vi "Compressor With Cylinder.vi"() -> ()   [LabVIEW 2013]
doc: "Compressor with Cylinder \n\nThis example shows how to control a compressor, extend and retract a cylinder, and optionally use a limit switch to retract automatically.\n\nThis example works with the NI 9403 module connected to a Digital Sidecar. The Digital Sidecar should have 12V applied to the WAGO connector. A SPIKE relay is used to turn the compressor on and off. The PWM type input on the SPIKE should be wired to RELAY 1 on the Digital Sidecar. The GND and 12V inputs on the SPIKE should get power from the battery through a 20A fuse on the Power Distribution Board. The M+ and M- outputs from the SPIKE should be wired to the compressor. Wire M+ to the red compressor wire, and M- to the black compressor wire. The Pressure Switch is wired to DIGITAL I/O 1. This input determines when the SPIKE relay gets energized to run the compressor. The Limit Switch is wired to DIGITAL I/O 2. It causes the cylinder to retract when the Auto Retract button is pressed.\n\nThis example also uses the Solenoid Breakout connected to the NI 9472 to control the SMC double solenoid valve. From the Solenoid Breakout, channel 1 is wired to terminal A on the valve, and channel 2 is wired to terminal B on the valve.\n\nRefer to the Pneumatics Manual for air connections. Your pneumatics setup should include a compressor, pressure switch, tank, regulator, valve, flow controls, cylinder, plug valve, etc.\n\nTo run this example you should have a pneumatic system with air pressure connected to the P input on the SMC double solenoid valve. The A output of the valve should be connected via a flow control to the backend of a cylinder. The B output of the valve should be connected via a flow control to the frontend of a cylinder. When the cylinder is extended, it should physically depress the Limit Switch.\n\nWith the VI running, pressing the Extend button will push the cylinder shaft out, and pressing the Retract button will pull it back. Notice that the Extend and Retract buttons have their Mechanical Action set to Latch When Pressed. This means they stay pressed (ON) until they are read by the program, then they return to the OFF position. This works because once the SMC solenoid valve is pulled one direction, it stays in that position until it is pulled in the opposite direction - it only needs to be momentarily energized. The Auto Retract button can be used to make the cylinder return automatically. With the Auto Retract button ON, pressing the Extend button will push the cylinder out, and it will retract when it hits the limit switch."
uses:
  <vilib>/Rock Robotics/WPI/Solenoid/WPI_SolenoidChannel.ctl
  <vilib>/Rock Robotics/SystemInterfaces/DIO/FPGA_DIOChannel.ctl
  <vilib>/Rock Robotics/SystemInterfaces/DIO/FPGA_DIORelayChannel.ctl
  <vilib>/Rock Robotics/SystemInterfaces/Typedef/FPGA_TypedefDigitalModule.ctl
  <vilib>/Rock Robotics/SystemInterfaces/Typedef/FPGA_TypedefSolenoidModule.ctl
  <vilib>/Rock Robotics/WPI/Solenoid/WPI_SolenoidValue.ctl
  <vilib>/Rock Robotics/WPI/Solenoid/WPI_SolenoidOpenDouble.vi
  <vilib>/Rock Robotics/WPI/Solenoid/WPI_SolenoidSetEnum.vi
panel:
  in  "CylinderAction":T1
  out "Compressor Running?":bool
  in  "Solenoid Module":T2
  out "Cylinder Limit":bool
  in  "Limit Switch Channel":T3=enum."DIO 2"
  in  "Retract Solenoid Channel":T4=enum."Solenoid 2"
  in  "Switch and Relay Module":T5
  in  "RelayChannel":T6
  in  "Pressure Switch Channel":T3
  in  "Extend Solenoid Channel":T4
  out "Compressor Enabled?":bool
  in  "stop":bool
  # "Set these inputs before running."
  # "These can be set while running."
  # "Output information."
  # "Wiring Diagram for Digital Sidecar connected to an NI 9403"
  # "when extended, the cylinder should depress this"
  # "Limit\nSwitch"
  # "(-)"
  # "B"
  # "A"
  # "8\n7\n6\n5\n4\n3\n2\n1"
  # "RELAY"
  # "Pressure\nSwitch"
  # "Connect\nPower\nHere"
  # "GND"
  # "M-"
  # "Connect\nCompressor\nHere"
  # "SPIKE"
  # "12V"
  # "M+"
  # "B"
  # "20A"
  # "fuse"
  # "SPIKE Relay"
  # "PWM cable"
  # "COM"
  # "NC"
  # "NO"
  # "NC"
  # "C"
  # "PWR"
  # "SIG"
  # "(-)"
  # "14\n13\n12\n11\n10\n9\n8\n7\n6\n5\n4\n3\n2\n1"
  # "DIGITAL I/O"
  # "Digital Sidecar"
  # "Wiring Diagram for Solenoid Breakout connected to an NI 9472"
  # "GND"
  # "SIG"
  # "8\n7\n6\n5\n4\n3\n2\n1"
  # "+"
  # "12V from\nbattery"
  # "-"
  # "tubing port for retract side of cylinder"
  # "tubing port for extend side of cylinder"
  # "\"power good\"\n  LED"
  # "SMC double solenoid valve"
  # "B"
  # "A"
  # "B"
  # "A"
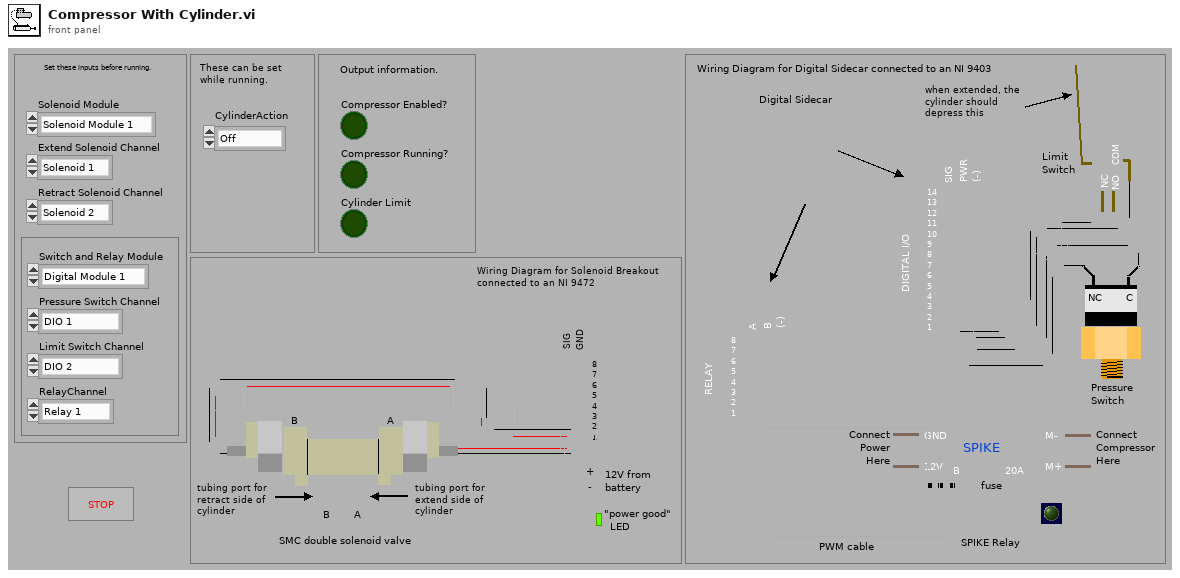
[diagram p1: front panel]
types:
  T1 = typedef "WPI_SolenoidValue.ctl" = enum16{"Off", "On", "Forward", "Reverse"}
  T2 = typedef "FPGA_TypedefSolenoidModule.ctl" = enum16{"Solenoid Module 1", "Solenoid Module 2"}
  T3 = typedef "FPGA_DIOChannel.ctl" = enum8{"DIO 1", "DIO 2", "DIO 3", "DIO 4", "DIO 5", "DIO 6", "DIO 7", "DIO 8", "DIO 9", "DIO 10", "DIO 11", "DIO 12", "DIO 13", "DIO 14", "Invalid"}
  T4 = typedef "WPI_SolenoidChannel.ctl" = enum8{"Solenoid 1", "Solenoid 2", "Solenoid 3", "Solenoid 4", "Solenoid 5", "Solenoid 6", "Solenoid 7", "Solenoid 8", "Invalid"}
  T5 = typedef "FPGA_TypedefDigitalModule.ctl" = enum16{"Digital Module 1", "Digital Module 2"}
  T6 = typedef "FPGA_DIORelayChannel.ctl" = enum8{"Relay 1", "Relay 2", "Relay 3", "Relay 4", "Relay 5", "Relay 6", "Relay 7", "Relay 8", "Invalid"}
  T7 = typedef "WPI_CompressorDevRef.ctl" = cluster{"DevStatus":errorcluster, "DigitalInputDevRef":T8, "RelayDevRef":T9}
  T8 = typedef "WPI_DigitalInputDevRef.ctl" = cluster{"DevStatus":errorcluster, "DIO Channel":T3, "Digital Module":T5}
  T9 = typedef "WPI_RelayDevRef.ctl" = cluster{"DevStatus":errorcluster, "Relay Channel":T6, "Digital Module":T5, "Relay Direction":T10}
  T10 = typedef "WPI_RelayDirection.ctl" = enum16{"Both directions", "Forward only", "Reverse only"}
  T11 = typedef "WPI_SolenoidDevRef.ctl" = cluster{"DevStatus":errorcluster, "Solenoid Module":T2, "Forward Solenoid Channel":T4, "Reverse Solenoid Channel":T4}
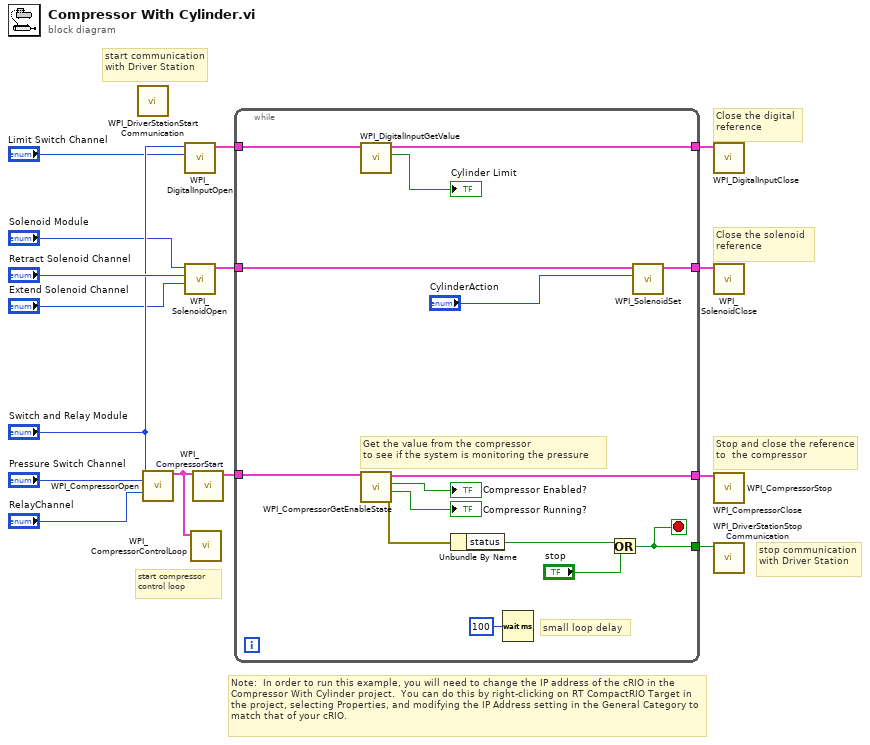
[diagram p0: block diagram]
diagram:
  # "start compressor control loop"
  # "Close the digital\nreference"
  # "Close the solenoid\nreference"
  # "stop communication with Driver Station"
  # "start communication with Driver Station"
  # "Note:  In order to run this example, you will need to change the IP address of the cRIO in the Compressor With Cylinder project.  You can do this by right-clicking on RT CompactRIO Target in the project, selecting Properties, and modifying the IP Address setting in the General Category to match that of your cRIO."
  # "Stop and close the reference to  the compressor"
  n1 = call <vilib>:"WPI_DriverStationStart Communication.vi"() -> ()  [unwired: 1 in, 11 out]
  n2 = call <vilib>:"WPI_CompressorOpen.vi"("Pressure Switch Digital Module (Module 1)"="Switch and Relay Module", "Pressure Switch DIO Channel"="Pressure Switch Channel", "Relay Channel"="RelayChannel") -> ("CompressorDevRef"=w1:T7)  [unwired: 2 in, 10 out]
  n3 = call <vilib>:"WPI_DigitalInputOpen.vi"("DIO Channel"="Limit Switch Channel", "Digital Module (Module 1)"="Switch and Relay Module") -> ("DigitalInputDevRef"=w7:T8)  [unwired: 1 in, 8 out]
  n4 = call-poly <vilib>:"WPI_SolenoidOpen.vi"("Reverse Solenoid Channel"="Extend Solenoid Channel", "Forward Solenoid Channel"="Retract Solenoid Channel", "Solenoid Module (Module 1)"="Solenoid Module") -> ("SolenoidDevRef"=w9:T11)  [unwired: 1 in, 7 out]
  n5 = call <vilib>:"WPI_CompressorControlLoop.vi"("CompressorDevRef"=w1) -> ()  [unwired: 11 in]
  n6 = call <vilib>:"WPI_CompressorStart.vi"("CompressorDevRef"=w1) -> ("CompressorDevRef"=w15:T7)  [unwired: 1 in, 9 out]
  n7 = while {
    tunnel: w15 -> [w31]
    tunnel: [w30] -> w14
    tunnel: [w28] -> w11
    tunnel: w9 -> [w23]
    tunnel: [w19] -> w10
    tunnel: w7 -> [w22]
    tunnel: [w21] -> w6
    stop <- w28 stop-if-true
    # "small loop delay"
    # "Get the value from the compressor \nto see if the system is monitoring the pressure"
    n8 = call <vilib>:"WPI_DigitalInputGetValue.vi"("DigitalInputDevRef"=w22) -> ("Value"=→"Cylinder Limit":bool, "DigitalInputDevRef"=w21:T8)  [unwired: 1 in, 8 out]
    n9 = call <vilib>:"WPI_CompressorGetEnableState.vi"("CompressorDevRef"=w31) -> ("error out"=w26:errorcluster, "Compressor Running"=→"Compressor Running?":bool, "Enabled"=→"Compressor Enabled?":bool, "CompressorDevRef"=w30:T7)  [unwired: 1 in, 6 out]
    n10 = Unbundle By Name(w26) -> ("status"=w25:bool)
    n11 = Wait (ms)(milliseconds to wait=u32 100) -> ()  [unwired: 1 out]
    n12 = Or(x=w25, y="stop") -> (x .or. y?=w28:bool)
    n13 = call-poly <vilib>:"WPI_SolenoidSet.vi"("Value"="CylinderAction", "SolenoidDevRef"=w23) -> ("SolenoidDevRef"=w19:T11)  [unwired: 1 in, 8 out]
  }
  n14 = call <vilib>:"WPI_DigitalInputClose.vi"("DigitalInputDevRef"=w6) -> ()  [unwired: 1 in, 10 out]
  n15 = call <vilib>:"WPI_SolenoidClose.vi"("SolenoidDevRef"=w10) -> ()  [unwired: 1 in, 10 out]
  n16 = call <vilib>:"WPI_CompressorStop.vi"("CompressorDevRef"=w14) -> ("CompressorDevRef"=w16:T7)  [unwired: 1 in, 9 out]
  n17 = call <vilib>:"WPI_CompressorClose.vi"("CompressorDevRef"=w16) -> ()  [unwired: 1 in, 10 out]
  n18 = call <vilib>:"WPI_DriverStationStop Communication.vi"("StopCommunication"=w11) -> ()  [unwired: 1 in, 10 out]
